vi "F Dwf Analog Out Play Data.vi"(7 "cdData":i32, 8 "error in (no error)":errorcluster, 9 "rgdData":dbl, 10 "idxChannel":i32, 11 "hdwf":i32) -> (0 "error out":errorcluster, 1 "rgdData out":dbl, 3 "function return":i32)   [LabVIEW 2019, in "Olasdwf.lvlib"]
doc: "DWFAPI int FDwfAnalogOutPlayData(HDWF hdwf, int idxChannel, double *rgdData, int cdData);"
uses:
  Olasdwf.lvlib
  Windows/System32/dwf.dll
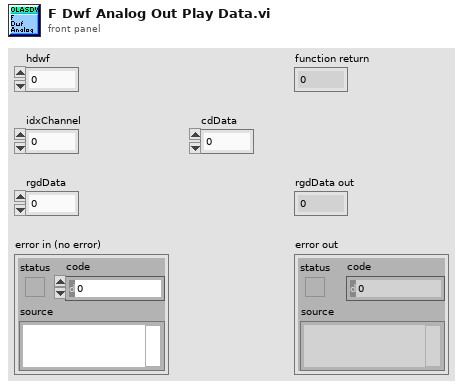
[diagram p1: front panel]
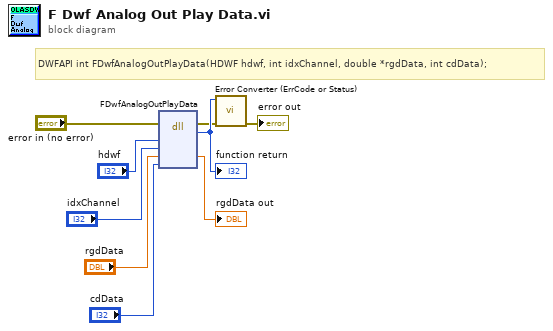
[diagram p0: block diagram]
diagram:
  # "DWFAPI int FDwfAnalogOutPlayData(HDWF hdwf, int idxChannel, double *rgdData, int cdData);"
  n1 = dll-call lib="C:/Windows/System32/dwf.*" fn="FDwfAnalogOutPlayData"(error in="error in (no error)", "hdwf"="hdwf", "idxChannel"="idxChannel", "rgdData"="rgdData", "cdData"="cdData") -> (error out=w2:errorcluster, w9:i32, "rgdData"=→"rgdData out":dbl)  [unwired: 5 in, 1 out]
  "function return" <- w9
  n2 = call "Error Converter (ErrCode or Status).vi"("error in (no error)"=w2, "error code"=w9) -> ("error out"=→"error out":errorcluster)  [unwired: 9 in]
